vi "auto.vi"() -> ()   [LabVIEW 2012, in "Mecanum Drive.lvrbt"]
uses:
  Mecanum Drive.lvrbt
  SubVIs/auto_drive_TYP.ctl
  SubVIs/State_Typ.ctl
  <vilib>/NXT/Hardware/Plugins/Tetrix DC Motor/TetrixDCMotorAddress.ctl
  <vilib>/NXT/Dual Mode Library/Waits/Wait_Num(msec).vi
  <vilib>/NXT/NXTIO Xnodes/NXTIONodeSubVIs/TETRIX IO Check Battery.vi
  <vilib>/NXT/NXTIO Xnodes/NXTIONodeSubVIs/TETRIX IO Stop DC Motors.vi
  <vilib>/NXT/Subs/LVHSConnector.ctl
  <vilib>/NXT/NXTIO Xnodes/AddressXNode/NXTIOAddress.xnode
  <vilib>/NXT/NXTIO Xnodes/NXTIOXNode/NXTIO.xnode
  <vilib>/NXT/LegoClasses/BrickReference/BrickReference.lvclass
panel:
  out "Enabled":bool
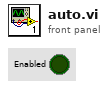
[diagram p1: front panel]
types:
  T1 = typedef "State_Typ.ctl" = enum16{"Move", "Check for Position 2", "Check for Position 3", "Stop"}
  T2 = typedef "auto_drive_TYP.ctl" = cluster{"Left X":i8, "Left Y":i8, "Right X":i8, "Power (100)":i8, "Wait (ms)":u32}
  T3 = typedef "TetrixDCMotorAddress.ctl" = i32
  T4 = typedef "LVHSConnector.ctl" = refnum<class "BrickReference.lvclass">
  T5 = cluster{"TetrixDCMotor":T3, "TetrixDCMotor 2":T3}
  T6 = cluster{"Direction (0-9)":i16, "Signal Strength (Array)":u8[]}
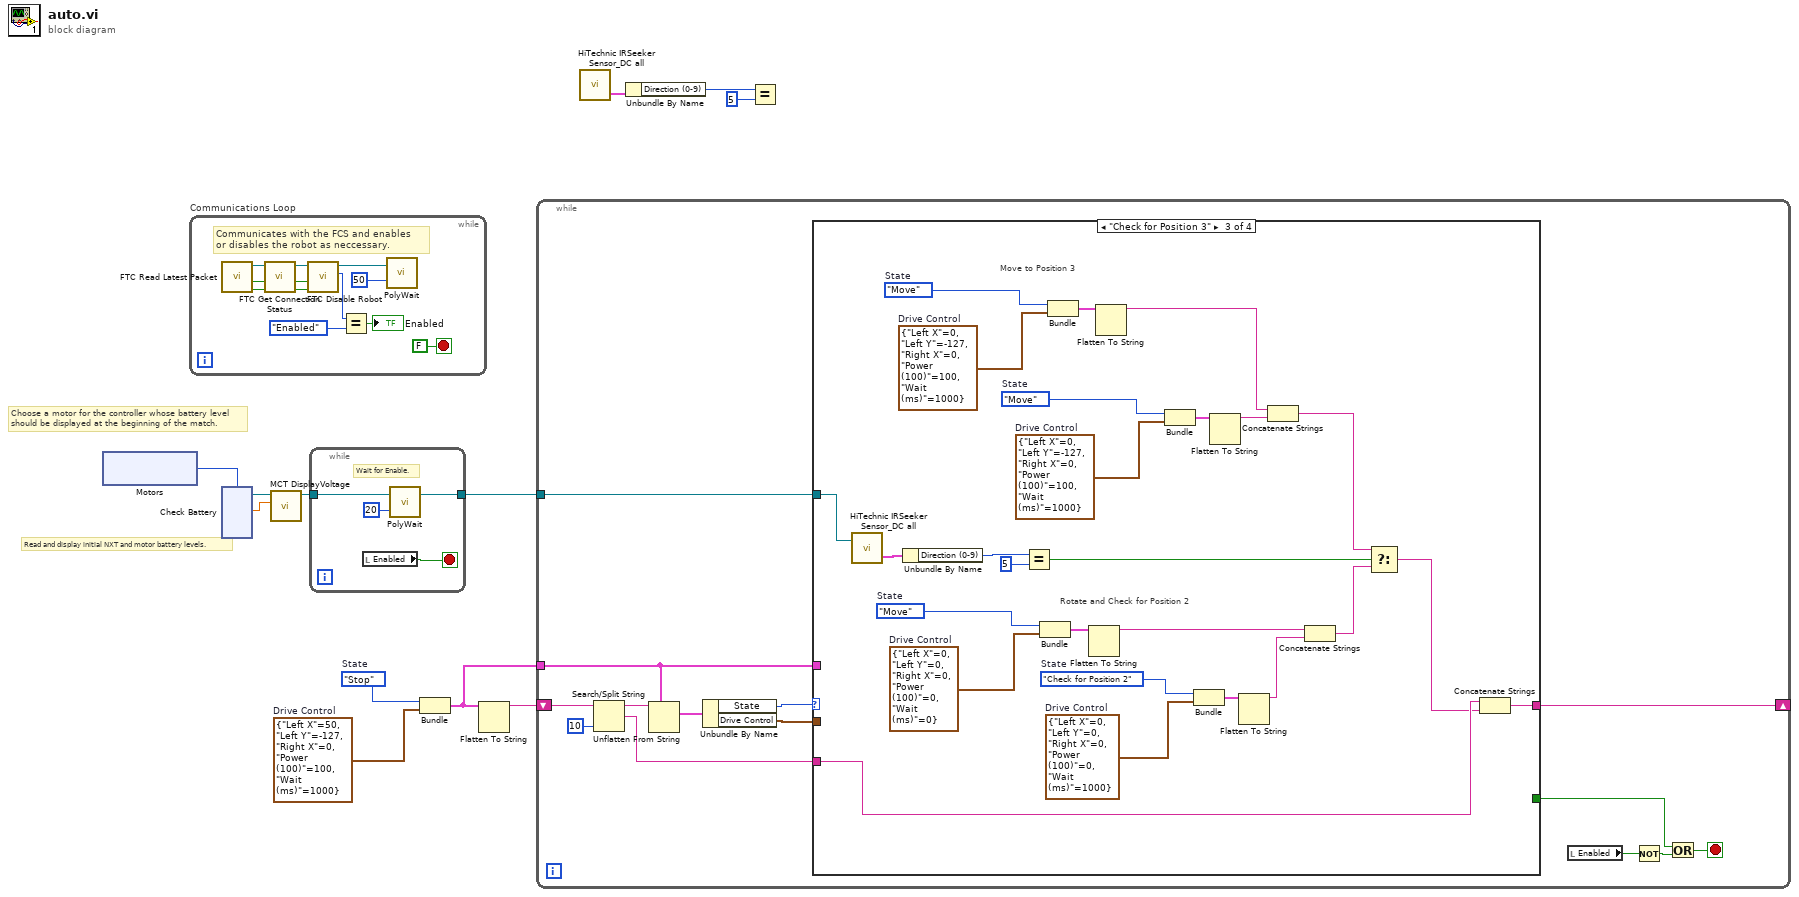
[diagram p0: block diagram]
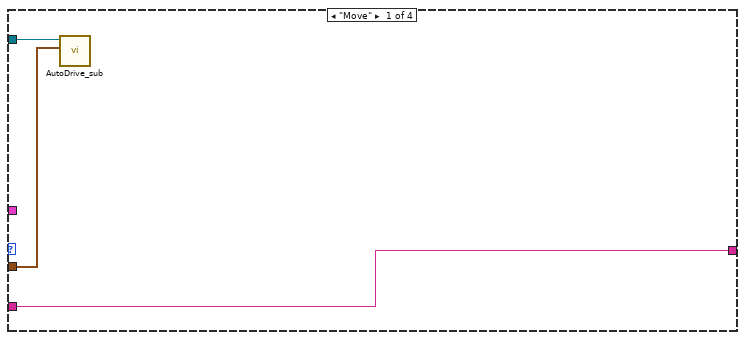
[diagram p2: hidden frame]
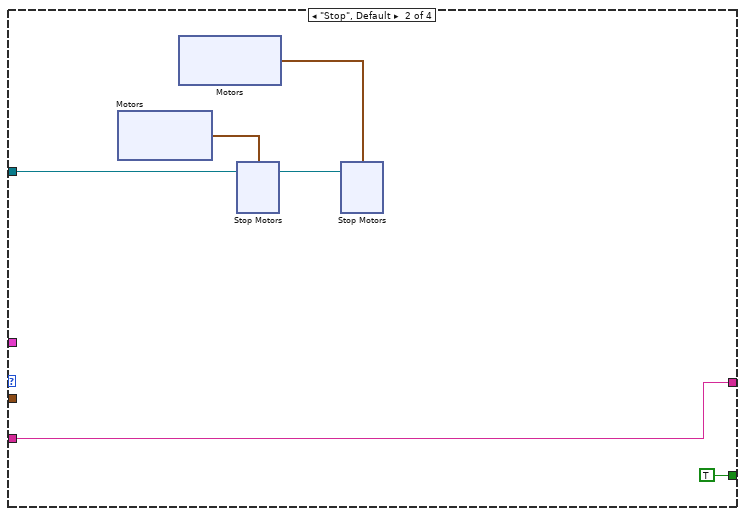
[diagram p3: hidden frame]
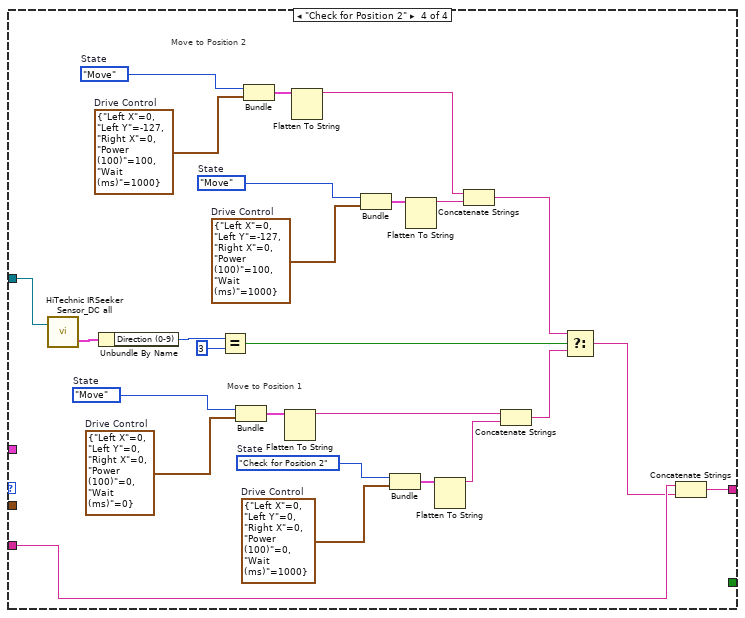
[diagram p4: hidden frame]
diagram:
  w4 = State_Typ."Stop"  # State
  w3 = T2 {"Left X"=50, "Left Y"=-127, "Right X"=0, "Power (100)"=100, "Wait (ms)"=1000}  # Drive Control
  # "Read and display initial NXT and motor battery levels."
  # "Choose a motor for the controller whose battery level \nshould be displayed at the beginning of the match."
  n1 = xnode "Motors"() -> ("Motor"=w9:T3)
  n2 = while "Communications Loop" {
    stop <- FALSE stop-if-true
    # "Communicates with the FCS and enables \nor disables the robot as neccessary."
    n3 = call <vilib>:"FTC Read Latest Packet.vi"() -> ("Packet Received?"=w22:bool, "Stopped?"=w21:bool, "NXT/EV3"=w24:T4)  [unwired: 6 in, 3 out]
    n4 = call <vilib>:"FTC Get Connection Status.vi"("Packet Received?"=w22, "Stopped?"=w21, "NXT/EV3"=w24) -> ("Online?"=w13:bool, "Stopped?"=w14:bool, "NXT/EV3"=w23:T4)  [unwired: 5 in]
    n5 = call <vilib>:"FTC Disable Robot.vi"("Online?"=w13, "Stopped?"=w14, "NXT/EV3"=w23) -> ("Enabled?"=w17:enum16{"Disabled", "Enabled"}, "NXT/EV3"=w19:T4)  [unwired: 3 in]
    n6 = Equal?(x=w17, y=enum16{"Disabled", "Enabled"}."Enabled") -> (x = y?=→"Enabled":bool)
    n7 = call-poly <vilib>:"PolyWait.vi"("Time (100 msec)"=u32 50 ("Time (msec)"), "NXT/EV3"=w19) -> ()  [unwired: 2 in, 1 out]
  }
  n8 = xnode "Check Battery"("Motors"=w9) -> ("Voltage 1"=w10:sgl, "NXT/EV3"=w12:T4)  [unwired: 1 in]
  n9 = call <vilib>:"MCT DisplayVoltage.vi"("Motor Voltage"=w10, "NXT/EV3"=w12) -> ("NXT/EV3"=w11:T4)  [unwired: 9 in]
  n10 = while {
    tunnel: [w26] -> w5
    tunnel: w11 -> [w25]
    stop <- w27 stop-if-true
    # "Wait for Enable."
    n11 = local read "Enabled"() -> (w27:bool)
    n12 = call-poly <vilib>:"PolyWait.vi"("Time (100 msec)"=u32 20 ("Time (msec)"), "NXT/EV3"=w25) -> ("NXT/EV3"=w26:T4)  [unwired: 2 in]
  }
  n13 = Bundle("State"=w4, "Drive Control"=w3) -> (w1:cluster{"State":T1, "Drive Control":T2})  [unwired: 1 in]
  n14 = Flatten To String(anything=w1) -> (data string=w2:string)  [unwired: 3 in, 2 out]
  n15 = while {
    tunnel: w5 -> [w42]
    shift-right: [w29] -> _
    shift-left: w2 -> [w37]
    tunnel: w1 -> [w31]
    stop <- w41 stop-if-true
    n16 = Search/Split String(string=w37, offset (0)=10 ("length (rest)")) -> (substring before match=w33:string, match + rest of string=w30:string)  [unwired: 1 in, 1 out]
    n17 = Unflatten From String(type=w31, binary string=w33) -> (value=w32:cluster{"State":T1, "Drive Control":T2})  [unwired: 3 in, 2 out]
    n18 = Unbundle By Name(w32) -> ("State"=w35:T1, "Drive Control"=w34:T2)
    n19 = case shown="\"Check for Position 3\"" w35 {
      tunnel: w42 -> [w45 w49 w86 w112]
      tunnel: [_ TRUE _ _] -> w40
      tunnel: w34 -> [w44 _ _ _]
      tunnel: w31 -> [_ _ _ _]
      tunnel: w30 -> [w43 w46 w66 w92]
      tunnel: [w43 w46 w65 w91] -> w29
      frame "Move" {
        n20 = call "AutoDrive_sub.vi"("Drive Control"=w44, "NXT/EV3"=w45) -> ()  [unwired: 9 in, 1 out]
      }
      frame "Stop", Default {
        n21 = xnode "Motors"() -> ("Motor"=w51:cluster{"TetrixDCMotor":T3, "TetrixDCMotor":T3})
        n22 = xnode "Motors"() -> ("Motor"=w50:cluster{"TetrixDCMotor":T3, "TetrixDCMotor":T3})
        n23 = xnode "Stop Motors"("Motors"=w51, "NXT/EV3"=w49) -> ("NXT/EV3"=w48:T4)
        n24 = xnode "Stop Motors"("Motors"=w50, "NXT/EV3"=w48) -> ()  [unwired: 1 out]
      }
      frame "Check for Position 3" {
        w71 = T2 {"Left X"=0, "Left Y"=0, "Right X"=0, "Power (100)"=0, "Wait (ms)"=1000}  # Drive Control
        w70 = State_Typ."Check for Position 2"  # State
        w79 = T2 {"Left X"=0, "Left Y"=-127, "Right X"=0, "Power (100)"=100, "Wait (ms)"=1000}  # Drive Control
        w80 = State_Typ."Move"  # State
        w81 = T2 {"Left X"=0, "Left Y"=0, "Right X"=0, "Power (100)"=0, "Wait (ms)"=0}  # Drive Control
        w82 = State_Typ."Move"  # State
        w84 = T2 {"Left X"=0, "Left Y"=-127, "Right X"=0, "Power (100)"=100, "Wait (ms)"=1000}  # Drive Control
        w83 = State_Typ."Move"  # State
        # "Move to Position 3"
        # "Rotate and Check for Position 2"
        n25 = call <vilib>:"HiTechnic IRSeeker Sensor_DC all.vi"("NXT/EV3"=w86) -> ("All Info"=w89:T6)  [unwired: 2 in, 1 out]
        n26 = Unbundle By Name(w89) -> ("Direction (0-9)"=w87:i16)
        n27 = Equal?(x=w87, y=i16 5) -> (x = y?=w85:bool)
        n28 = Bundle("State"=w82, "Drive Control"=w81) -> (w73:cluster{"State":T1, "Drive Control":T2})  [unwired: 1 in]
        n29 = Bundle("State"=w83, "Drive Control"=w84) -> (w78:cluster{"State":T1, "Drive Control":T2})  [unwired: 1 in]
        n30 = Flatten To String(anything=w73) -> (data string=w68:string)  [unwired: 3 in, 2 out]
        n31 = Flatten To String(anything=w78) -> (data string=w75:string)  [unwired: 3 in, 2 out]
        n32 = Bundle("State"=w80, "Drive Control"=w79) -> (w77:cluster{"State":T1, "Drive Control":T2})  [unwired: 1 in]
        n33 = Bundle("State"=w70, "Drive Control"=w71) -> (w72:cluster{"State":T1, "Drive Control":T2})  [unwired: 1 in]
        n34 = Flatten To String(anything=w77) -> (data string=w76:string)  [unwired: 3 in, 2 out]
        n35 = Flatten To String(anything=w72) -> (data string=w69:string)  [unwired: 3 in, 2 out]
        n36 = Concatenate Strings(w75, w76) -> (w74:string)
        n37 = Concatenate Strings(w68, w69) -> (w67:string)
        n38 = Select(t=w74, s=w85, f=w67) -> (s? t:f=w64:string)
        n39 = Concatenate Strings(w66, w64) -> (w65:string)
      }
      frame "Check for Position 2" {
        w97 = T2 {"Left X"=0, "Left Y"=0, "Right X"=0, "Power (100)"=0, "Wait (ms)"=1000}  # Drive Control
        w96 = State_Typ."Check for Position 2"  # State
        w105 = T2 {"Left X"=0, "Left Y"=-127, "Right X"=0, "Power (100)"=100, "Wait (ms)"=1000}  # Drive Control
        w106 = State_Typ."Move"  # State
        w107 = T2 {"Left X"=0, "Left Y"=0, "Right X"=0, "Power (100)"=0, "Wait (ms)"=0}  # Drive Control
        w108 = State_Typ."Move"  # State
        w110 = T2 {"Left X"=0, "Left Y"=-127, "Right X"=0, "Power (100)"=100, "Wait (ms)"=1000}  # Drive Control
        w109 = State_Typ."Move"  # State
        # "Move to Position 1"
        # "Move to Position 2"
        n40 = call <vilib>:"HiTechnic IRSeeker Sensor_DC all.vi"("NXT/EV3"=w112) -> ("All Info"=w115:T6)  [unwired: 2 in, 1 out]
        n41 = Unbundle By Name(w115) -> ("Direction (0-9)"=w113:i16)
        n42 = Equal?(x=w113, y=i16 3) -> (x = y?=w111:bool)
        n43 = Bundle("State"=w108, "Drive Control"=w107) -> (w99:cluster{"State":T1, "Drive Control":T2})  [unwired: 1 in]
        n44 = Bundle("State"=w109, "Drive Control"=w110) -> (w104:cluster{"State":T1, "Drive Control":T2})  [unwired: 1 in]
        n45 = Flatten To String(anything=w99) -> (data string=w94:string)  [unwired: 3 in, 2 out]
        n46 = Flatten To String(anything=w104) -> (data string=w101:string)  [unwired: 3 in, 2 out]
        n47 = Bundle("State"=w106, "Drive Control"=w105) -> (w103:cluster{"State":T1, "Drive Control":T2})  [unwired: 1 in]
        n48 = Bundle("State"=w96, "Drive Control"=w97) -> (w98:cluster{"State":T1, "Drive Control":T2})  [unwired: 1 in]
        n49 = Flatten To String(anything=w103) -> (data string=w102:string)  [unwired: 3 in, 2 out]
        n50 = Flatten To String(anything=w98) -> (data string=w95:string)  [unwired: 3 in, 2 out]
        n51 = Concatenate Strings(w101, w102) -> (w100:string)
        n52 = Concatenate Strings(w94, w95) -> (w93:string)
        n53 = Select(t=w100, s=w111, f=w93) -> (s? t:f=w90:string)
        n54 = Concatenate Strings(w92, w90) -> (w91:string)
      }
    }
    n55 = local read "Enabled"() -> (w39:bool)
    n56 = Not(x=w39) -> (.not. x?=w38:bool)
    n57 = Or(x=w40, y=w38) -> (x .or. y?=w41:bool)
  }
  n58 = call <vilib>:"HiTechnic IRSeeker Sensor_DC all.vi"() -> ("All Info"=w6:T6)  [unwired: 3 in, 1 out]
  n59 = Unbundle By Name(w6) -> ("Direction (0-9)"=w7:i16)
  n60 = Equal?(x=w7, y=i16 5) -> ()  [unwired: 1 out]
